vi "testProcessEvent.vi"(8 "error in (no error)":errorcluster) -> (0 "error out":errorcluster)   [LabVIEW 2018]
doc: "Test the processEvent.vi."
uses:
  src/TcpServer/TcpServer.lvclass
  src/TcpServer/TcpServer.lvclass/TcpServer.ctl
  src/TcpServerBase/typedef/tcpPacketTypeDef.ctl
  <vilib>/addons/_JKI Toolkits/Caraya/classes/Assert/Assert Equal Value_Variant.vi
  src/TcpServerCmd/TcpServerCmd.lvclass
  <vilib>/addons/_JKI Toolkits/Caraya/classes/Test/Test.lvclass
  <vilib>/addons/_JKI Toolkits/Caraya/classes/Assert/Assert.lvclass
  src/TcpServerBase/TcpServerBase.lvclass
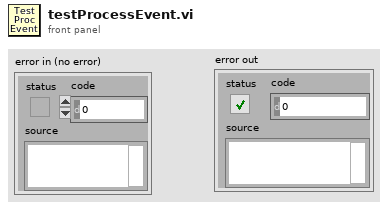
[diagram p1: front panel]
types:
  T1 = typedef "TcpServerBase.lvclass/tcpPacketTypeDef.ctl" = cluster{"packet":string, "firstPacket":bool, "firstConnection":bool}
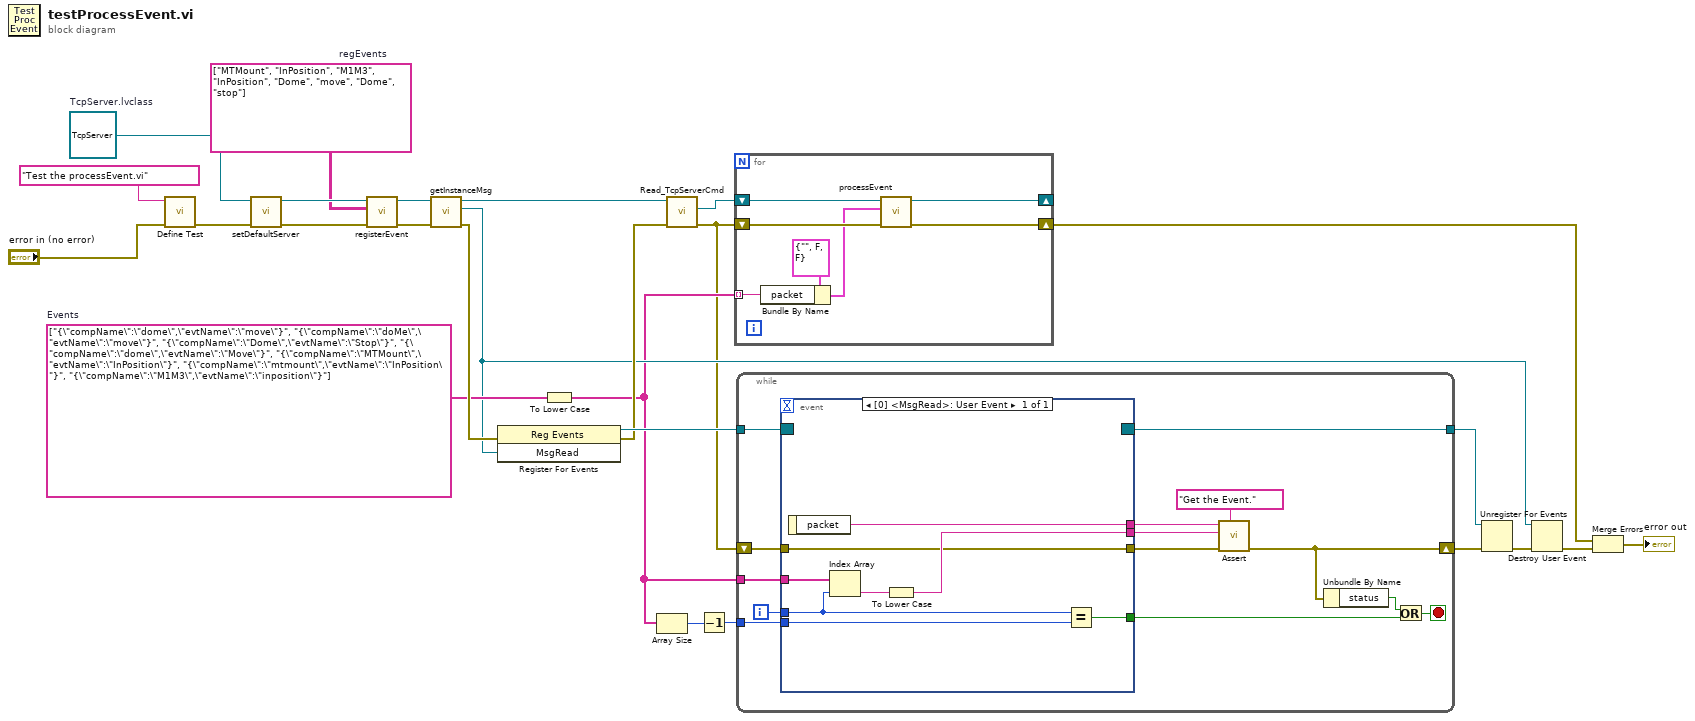
[diagram p0: block diagram]
diagram:
  w17 = string[][] [["MTMount", "InPosition"], ["M1M3", "InPosition"], ["Dome", "move"], ["Dome", "stop"]]  # regEvents
  w12 = string[] ["{\"compName\":\"dome\",\"evtName\":\"move\"}", "{\"compName\":\"doMe\",\"evtName\":\"move\"}", "{\"compName\":\"Dome\",\"evtName\":\"Stop\"}", "{\"compName\":\"dome\",\"evtName\":\"Move\"}", "{\"compName\":\"MTMount\",\"evtName\":\"InPosition\"}", "{\"compName\":\"mtmount\",\"evtName\":\"InPosition\"}", "{\"compName\":\"M1M3\",\"evtName\":\"inposition\"}"]  # Events
  w23 = refnum<class "TcpServer.lvclass"> refnum  # TcpServer.lvclass
  n1 = call <vilib>:"Define Test.vi"("error in (no error)"="error in (no error)", "Label (VI Title)"="Test the processEvent.vi") -> ("error out"=w25:errorcluster)  [unwired: 9 in]
  n2 = call "setDefaultServer.vi"("error in (no error)"=w25, "TcpServer.lvclass"=w23) -> ("error out"=w22:errorcluster, "tcpServer out"=w18:refnum<class "TcpServer.lvclass">)  [unwired: 8 in]
  n3 = call "registerEvent.vi"("error in (no error)"=w22, "regEvent"=w17, "tcpServer in"=w18) -> ("error out"=w19:errorcluster, "tcpServer out"=w15:refnum<class "TcpServer.lvclass">)  [unwired: 7 in]
  n4 = call "getInstanceMsg.vi"("error in (no error)"=w19, "tcpServer in"=w15) -> ("error out"=w14:errorcluster, "MsgRead"=w7:refnum<user-event>, "tcpServer out"=w2:refnum<class "TcpServer.lvclass">)  [unwired: 6 in, 1 out]
  n5 = register-events(error in=w14, w7) -> (reference out=w13:refnum<event-registration>, error out=w11:errorcluster)  [unwired: 1 in]
  n6 = To Lower Case(string=w12) -> (all lower case string=w4:string[])
  n7 = Array Size(array=w4) -> (size(s)=w16:i32)
  n8 = call "Read_TcpServerCmd.vi"("error in (no error)"=w11, "TcpServer in"=w2) -> ("error out"=w3:errorcluster, "TcpServerCmd.lvclass"=w1:refnum<class "TcpServerCmd.lvclass">)  [unwired: 7 in, 1 out]
  n9 = Decrement(x=w16) -> (x-1=w5:i32)
  n10 = for {
    tunnel: w4 -> [w29] mode=indexing
    shift-right: [w27] -> _
    shift-left: w1 -> [w31]
    shift-right: [w28] -> w20
    shift-left: w3 -> [w33]
    n11 = Bundle By Name(cluster=T1 {"packet"="", "firstPacket"=FALSE, "firstConnection"=FALSE} ("packetConnID"), "packet"=w29) -> (w30:T1)
    n12 = call "processEvent.vi"("error in (no error)"=w33, "tcpPacket"=w30, "tcpServerCmd in"=w31) -> ("error out"=w28:errorcluster, "tcpServerCmd out"=w27:refnum<class "TcpServerCmd.lvclass">)  [unwired: 7 in]
  }
  n13 = while {
    tunnel: w13 -> [w46]
    tunnel: w4 -> [w45]
    shift-right: [w34] -> w10
    shift-left: w3 -> [w44]
    tunnel: [w43] -> w9
    tunnel: w5 -> [w42]
    i -> [w47]
    stop <- w40 stop-if-true
    n14 = event shown="[0] <MsgRead>: User Event" {
      selector: w46 -> [_]
      dyn-events: [_] -> w43
      timeout: _ -> [_]
      tunnel: w47 -> [w52]
      tunnel: [w55] -> w39
      tunnel: w45 -> [w54]
      tunnel: w44 -> [w48]
      tunnel: w42 -> [w51]
      tunnel: [w50] -> w37
      tunnel: [w49] -> w36
      tunnel: [w48] -> w35
      event User Event {
        n15 = event-data() -> ("packet"=w50:string)  [unwired: 1 in]
        n16 = Index Array(array=w54, index=w52) -> (element=w53:string)
        n17 = To Lower Case(string=w53) -> (all lower case string=w49:string)
        n18 = Equal?(x=w52, y=w51) -> (x = y?=w55:bool)
      }
    }
    n19 = call-poly <vilib>:"Assert.vi"("Label"="Get the Event.", "error in (no error)"=w35, "Y"=w36, "X"=w37) -> ("error out"=w34:errorcluster)  [unwired: 7 in]
    n20 = Unbundle By Name(w34) -> ("status"=w41:bool)
    n21 = Or(x=w41, y=w39) -> (x .or. y?=w40:bool)
  }
  n22 = Unregister For Events(event registration refnum=w9, error in=w10) -> (error out=w8:errorcluster)
  n23 = Destroy User Event(user event=w7, error in=w8) -> (error out=w6:errorcluster)
  n24 = Merge Errors(w20, w6) -> (→"error out":errorcluster)
